vi "UTILITY Aquire Semaphore.vi"(8 "error in (no error)":errorcluster, 10 "Debug":bool, 11 "Refnum in":T1) -> (0 "error out":errorcluster, 2 "Local?":bool, 3 "Refnum out":T1)   [LabVIEW 2016]
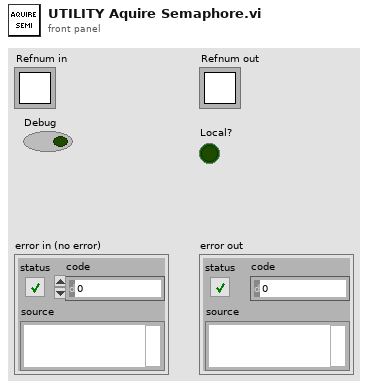
[diagram p1: front panel]
types:
  T1 = typedef "Semaphore RefNum" = refnum<k1>
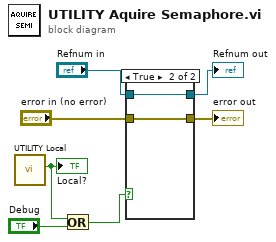
[diagram p0: block diagram]
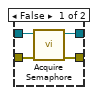
[diagram p2: hidden frame]
diagram:
  n1 = call "UTILITY Local.vi"() -> ("Local?"=w3:bool)  [unwired: 11 in]
  "Local?" <- w3
  n2 = Or(x=w3, y="Debug") -> (x .or. y?=w1:bool)
  n3 = case shown="True" w1 {
    tunnel: "error in (no error)" -> [w11 w13]
    tunnel: [w10 w13] -> w7
    tunnel: [w9 w12] -> w5
    tunnel: "Refnum in" -> [w8 w12]
    frame False {
      n4 = call <vilib>:"Acquire Semaphore.vi"("error in (no error)"=w11, "semaphore"=w8) -> ("error out"=w10:errorcluster, "semaphore out"=w9:T1)  [unwired: 3 in, 1 out]
    }
    frame True {
    }
  }
  "error out" <- w7
  "Refnum out" <- w5
